vi "HAL Camera specifications globals.vi"() -> ()   [LabVIEW 2011]
panel:
  out "Buffer":T1
  out "Camera Handle":u32
  in  "Camera Name":string="Orca Flash 4.0"
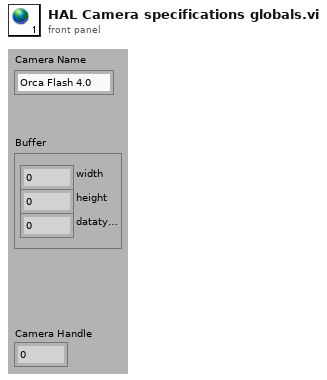
[diagram p1: front panel]
types:
  T1 = cluster{"width":u32, "height":u32, "datatype":u32}
diagram:
